vi "SetCurrent.vi"(2 "error out 2":errorcluster, 3 "string":string, 4 "reference out 2":refnum<visa-resource-name>) -> (0 "error out":errorcluster, 1 "reference out":refnum<visa-resource-name>)   [LabVIEW 2009]
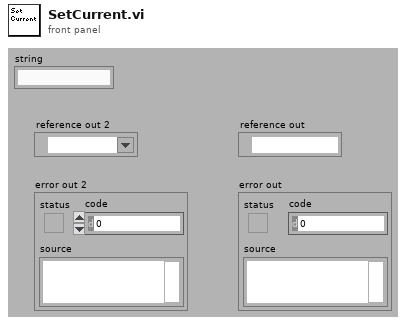
[diagram p1: front panel]
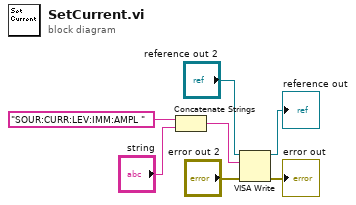
[diagram p0: block diagram]
diagram:
  n1 = Concatenate Strings("SOUR:CURR:LEV:IMM:AMPL " ("write buffer"), "string") -> (w1:string)
  n2 = VISA Write(VISA resource name="reference out 2", write buffer=w1, error in (no error)="error out 2") -> (VISA resource name out=→"reference out":refnum<visa-resource-name>, error out=→"error out":errorcluster)  [unwired: 1 out]
